vi "Measure JV curve.vi"(4 "Skip pixel?":bool, 6 "Scan settings":T1={"J-V scan"=TRUE, "J-t scan"=FALSE, "Min voltage (V)"=0.0, "Max voltage (V)"=1.4, "Step (V)"=0.01, "Measurement delay (ms)"=10.0, "1st scan FB-SC"=TRUE, "Inverted structure"=FALSE, "Stabilisation time (s)"=0.0, "Stabilisation mode"=0, "Stabilisation value (V or A) "=0.0, "Step time (s)"=1.0, "Integration time"=0, "Repeat light scans"=FALSE, "Stabilisation in the dark?"=FALSE, "J-t Min (V)"=0.0, "J-t Max (V)"=1.4, "J-t Step (V)"=0.01, "Max. power stabilisation"=FALSE, "J-t 1st scan FB-SC"=TRUE, "J-t Inverted structure"=FALSE, "Max power tracking"=FALSE, "Vmp (V)"=0.7, "Total stabilisation time (s)"=100.0, "J-t best pixel only"=0, "Max power best pixel only"=0, "Vmp from J-V scan"=FALSE, "Intensity dependence"=FALSE, "P dep best pixel only"=0, "External quantum efficiency"=FALSE, "EQE best pixel only"=0, "WL min (nm)"=300.0, "WL max (nm)"=900.0, "WL step (nm)"=5.0, "Wait (ms)"=100.0, "No. of repeat scans"=2.0, "Only repeat for best pixel"=0, "Chopper Freq. min (Hz)"=90.0, "Time Constant min (s)"=2.0, "Stabilisation time step (s)"=1.0, "Illumination conditions"=2, "Scan rate min (V/s)"=0.1, "Scan rate max (V/s)"=1.0, "No. of scan rate steps"=1.0, "Scan rate voltage step priority"=FALSE, "Scan rate measurement delay priority"=FALSE, "J-t Illumination conditions"=0, "Chopper Freq. max (Hz)"=200.0, "No. of freq. steps"=1.0, "Time Constant max (s)"=2.0, "No. of t const. steps"=1.0, "White bias min (no. of suns)"=0.1, "White bias max (no. of suns)"=1.0, "No. of white bias steps"=1.0, "Repeat EQE scans"=FALSE, "No. of EQE scans"=2.0, "Max P stab. Specific voltage"=FALSE} {"No. of EQE scans" min=1.0 step=1.0; "No. of white bias steps" min=1.0 step=1.0; "No. of t const. steps" min=1.0 step=1.0; "Time Constant max (s)" items=["0.01s", "0.03s", "0.1s", "0.3s", "1s", "3s"]; "No. of freq. steps" min=1.0 step=1.0; "J-t Illumination conditions" items=["Light only", "Dark only", "Light then dark", "Dark then light"]; "No. of scan rate steps" min=1.0 step=1.0; "Illumination conditions" items=["Light only", "Dark only", "Light then dark", "Dark then light", "Light then dark then light", "Dark then light then dark"]; "Time Constant min (s)" items=["0.01s", "0.03s", "0.1s", "0.3s", "1s", "3s"]; "Only repeat for best pixel" items=["only for best pixel", "for best 2 pixels", "for best 3 pixels", "for best 4 pixels", "for best 5 pixels", "for best 6 pixels", "for best 7 pixels", "for all pixels"]; "No. of repeat scans" min=1.0 step=1.0; "EQE best pixel only" items=["only the best pixel", "the best 2 pixel", "the best 3 pixel", "the best 4 pixel", "the best 5 pixel", "the best 6 pixel", "the best 7 pixel", "all pixels"]; "P dep best pixel only" items=["only the best pixel", "the best 2 pixels", "the best 3 pixels", "the best 4 pixels", "the best 5 pixels", "the best 6 pixels", "the best 7 pixels", "all pixels"]; "Max power best pixel only" items=["only the best pixel", "the best 2 pixels", "the best 3 pixels", "the best 4 pixels", "the best 5 pixels", "the best 6 pixels", "the best 7 pixels", "all pixels"]; "J-t best pixel only" items=["only the best pixel", "the best 2 pixels", "the best 3 pixels", "the best 4 pixels", "the best 5 pixels", "the best 6 pixels", "the best 7 pixels", "all pixels"]; "Integration time" items=["Fast", "Normal", "High Accuracy"]; "Stabilisation mode" items=["V", "I"]; "Measurement delay (ms)" min=10.0}, 7 "Cell details cluster":T3={"Cell Position"=16, "Cell Label"="", "Pixel to measure"=0, "Area (cm^2)"=0.126, "Variable"="", "Variable value"="", "Scan settings in queue"=0, "Light or dark"="", "Measurement type"=""} {"Pixel to measure" items=["All", "1", "2", "3", "4", "5", "6", "7", "8"]}, 8 "Intensity (no. of suns)":string, 9 "Scan rate (V/s)":dbl, 10 "Experiment Title":string, 11 "User Name":string) -> (0 "Log Table":string[][](table), 2 "File path for master log":path, 3 "JV Curve":cluster{"Y":dbl[], "Y":dbl[]}[](graph))   [LabVIEW 2011]
uses:
  TypeDefs/Scan settings.ctl
  TypeDefs/Settings Boolean.ctl
  TypeDefs/NPLC for JV scan.ctl
  <instrlib>/keithley_24xx/Keithley 24XX/Public/Data/Read (Single Point).vi
  <instrlib>/keithley_24xx/Keithley 24XX/Keithley 24XX.lvlib
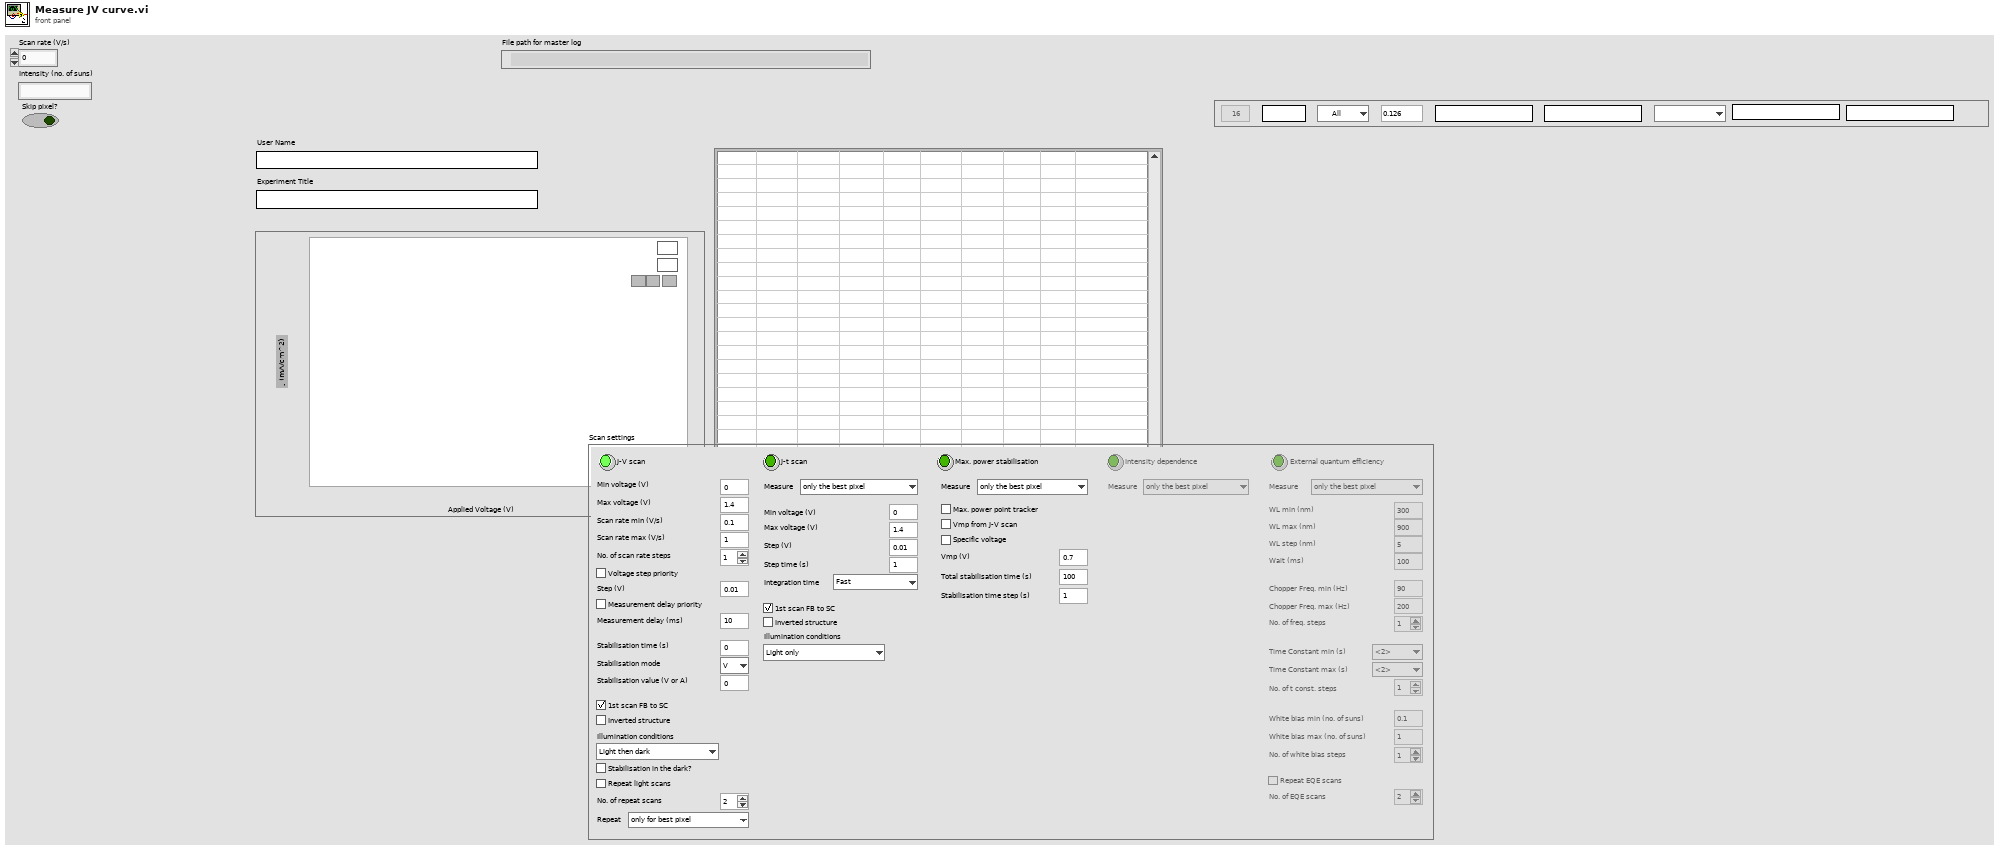
[diagram p1: front panel]
types:
  T1 = typedef "Scan settings.ctl" = cluster{"J-V scan":T2, "J-t scan":bool, "Min voltage (V)":dbl, "Max voltage (V)":dbl, "Step (V)":dbl, "Measurement delay (ms)":dbl, "1st scan FB-SC":bool, "Inverted structure":bool, "Stabilisation time (s)":dbl, "Stabilisation mode":u16, "Stabilisation value (V or A) ":dbl, "Step time (s)":dbl, "Integration time":u16, "Repeat light scans":bool, "Stabilisation in the dark?":bool, "J-t Min (V)":dbl, "J-t Max (V)":dbl, "J-t Step (V)":dbl, "Max. power stabilisation":bool, "J-t 1st scan FB-SC":bool, "J-t Inverted structure":bool, "Max power tracking":bool, "Vmp (V)":dbl, "Total stabilisation time (s)":dbl, "J-t best pixel only":u16, "Max power best pixel only":u16, "Vmp from J-V scan":bool, "Intensity dependence":bool, "P dep best pixel only":u16, "External quantum efficiency":bool, "EQE best pixel only":u16, "WL min (nm)":dbl, "WL max (nm)":dbl, "WL step (nm)":dbl, "Wait (ms)":dbl, "No. of repeat scans":dbl, "Only repeat for best pixel":u16, "Chopper Freq. min (Hz)":dbl, "Time Constant min (s)":dbl, "Stabilisation time step (s)":dbl, "Illumination conditions":u16, "Scan rate min (V/s)":dbl, "Scan rate max (V/s)":dbl, "No. of scan rate steps":dbl, "Scan rate voltage step priority":bool, "Scan rate measurement delay priority":bool, "J-t Illumination conditions":u16, "Chopper Freq. max (Hz)":dbl, "No. of freq. steps":dbl, "Time Constant max (s)":dbl, "No. of t const. steps":dbl, "White bias min (no. of suns)":dbl, "White bias max (no. of suns)":dbl, "No. of white bias steps":dbl, "Repeat EQE scans":bool, "No. of EQE scans":dbl, "Max P stab. Specific voltage":bool}
  T2 = typedef "Settings Boolean.ctl" = bool
  T3 = cluster{"Cell Position":i32, "Cell Label":string, "Pixel to measure":u16, "Area (cm^2)":dbl, "Variable":string, "Variable value":string, "Scan settings in queue":u16, "Light or dark":string, "Measurement type":string}
  T4 = typedef "NPLC for JV scan.ctl" = dbl
  T5 = typedef "imagedata.ctl" = cluster{"image type":i32, "image depth":i32, "image":u8[], "mask":u8[], "colors":u32[], "Rectangle":cluster{"left":i16, "top":i16, "right":i16, "bottom":i16}}
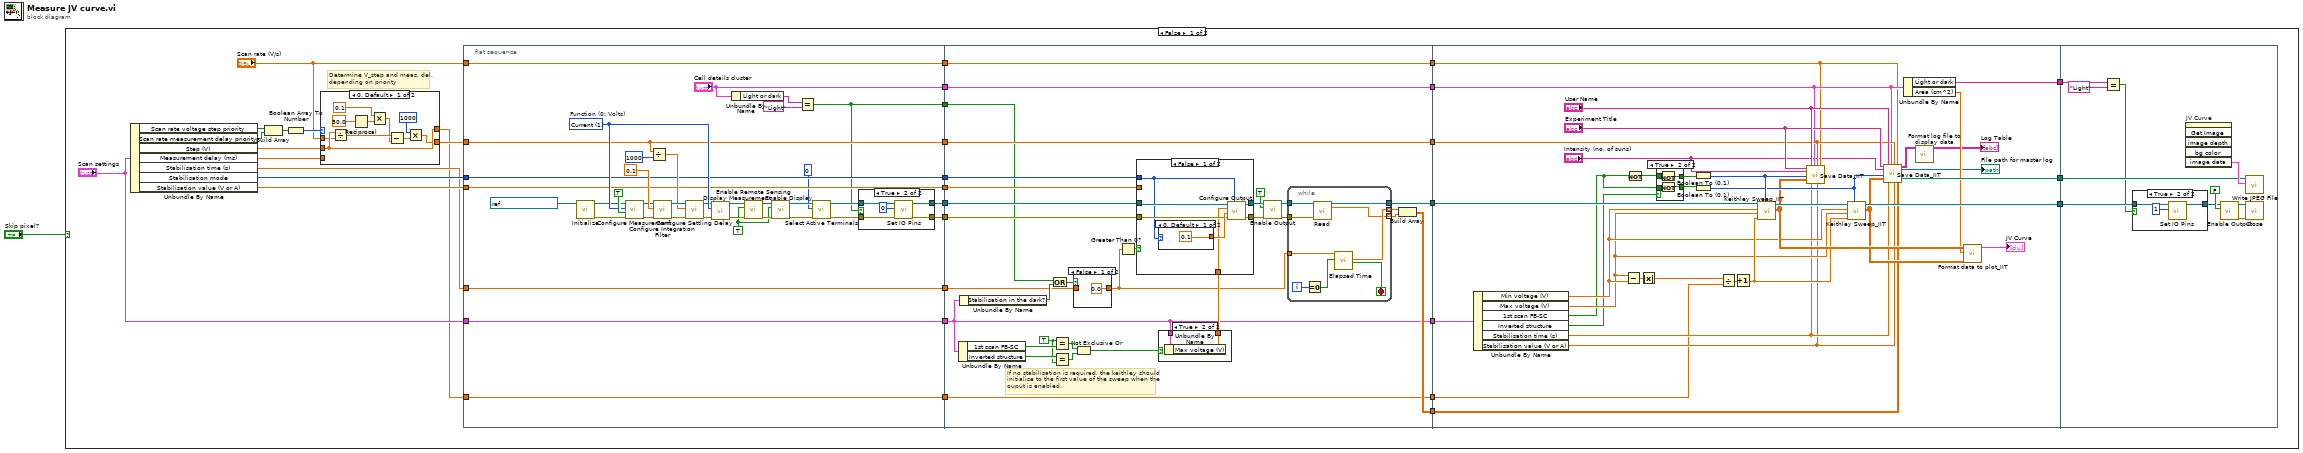
[diagram p0: block diagram]
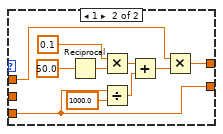
[diagram p2: hidden frame]
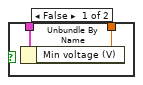
[diagram p5: hidden frame]
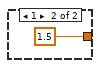
[diagram p6: hidden frame]
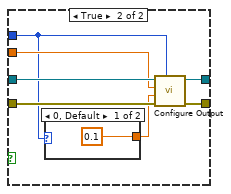
[diagram p7: hidden frame]
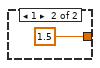
[diagram p8: hidden frame]
diagram:
  n1 = case shown="False" "Skip pixel?" {
    frame False {
      # "Determine V_step and meas. del.\ndepending on priority"
      n2 = Unbundle By Name("Scan settings") -> ("Scan rate voltage step priority"=w9:bool, "Scan rate measurement delay priority"=w8:bool, "Step (V)"=w3:dbl, "Measurement delay (ms)"=w5:dbl, "Stabilisation time (s)"=w11:dbl, "Stabilisation mode"=w13:u16, "Stabilisation value (V or A)"=w14:dbl)
      n3 = Build Array(w9, w8) -> (w10:bool[])
      n4 = Boolean Array To Number(Boolean array=w10) -> (number=w7:u32)
      n5 = case shown="0, Default" w7 {
        tunnel: [w39 w51] -> w6
        tunnel: w5 -> [_ w51]
        tunnel: "Scan rate (V/s)" -> [w36 w47]
        tunnel: [w45 w46] -> w4
        tunnel: w3 -> [w45 _]
        frame 0, Default {
          n6 = Divide(x=w45, y=w36) -> (x/y=w41:dbl)
          n7 = Reciprocal(x=50.0) -> (1/x=w43:dbl)
          n8 = Multiply(x=T4 0.1, y=w43) -> (x*y=w40:T4)
          n9 = Subtract(x=w41, y=w40) -> (x-y=w38:T4)
          n10 = Multiply(x=1000, y=w38) -> (x*y=w39:T4)
        }
        frame 1 {
          n11 = Reciprocal(x=50.0) -> (1/x=w54:dbl)
          n12 = Multiply(x=T4 0.1, y=w54) -> (x*y=w52:T4)
          n13 = Divide(x=w51, y=1000.0) -> (x/y=w49:dbl)
          n14 = Add(x=w52, y=w49) -> (x+y=w48:T4)
          n15 = Multiply(x=w47, y=w48) -> (x*y=w46:T4)
        }
      }
      n16 = flat-sequence {
        tunnel: [w73] -> w35
        tunnel: [w66] -> w34
        tunnel: [w67] -> w33
        tunnel: w14 -> [w73]
        tunnel: [w72] -> w32
        tunnel: w13 -> [w72]
        tunnel: [w71] -> w31
        tunnel: w11 -> [w71]
        tunnel: w6 -> [w70]
        tunnel: [w70] -> w30
        tunnel: [w69] -> w29
        tunnel: "Scan settings" -> [w69]
        tunnel: ["Cell details cluster"] -> w28
        tunnel: [w58] -> w27
        tunnel: [w57] -> w26
        tunnel: w4 -> [w57]
        tunnel: [w56] -> w25
        tunnel: "Scan rate (V/s)" -> [w56]
        tunnel: w35 -> [w119]
        tunnel: w34 -> [w127]
        tunnel: w33 -> [w128]
        tunnel: [w123] -> w24
        tunnel: [w120] -> w23
        tunnel: w32 -> [w116]
        tunnel: w31 -> [w102]
        tunnel: [w118] -> w22
        tunnel: w30 -> [w118]
        tunnel: [w107] -> w21
        tunnel: w29 -> [w107]
        tunnel: [w117] -> w20
        tunnel: w28 -> [w117]
        tunnel: w27 -> [w105]
        tunnel: [w101] -> w19
        tunnel: w26 -> [w101]
        tunnel: [w100] -> w18
        tunnel: w25 -> [w100]
        tunnel: [w192] -> w17
        tunnel: [w185] -> w16
        tunnel: w24 -> [w199]
        tunnel: w23 -> [w184]
        tunnel: w22 -> [w181]
        tunnel: w21 -> [w180]
        tunnel: w20 -> [w174]
        tunnel: [w173] -> w15
        tunnel: w19 -> [w166]
        tunnel: w18 -> [w165]
        tunnel: w17 -> [w210]
        tunnel: w16 -> [w211]
        tunnel: w15 -> [w206]
        frame #0 {
          w74 = TRUE ("Enable Output (T: Enable)")
          w87 = u16 1 items=["Volts", "Current", "Resistance"]  # Function (0: Volts)
          n17 = call <instrlib>:"Initialize.vi"("VISA resource name"=refnum<visa-resource-name> "GPIB0::24::INSTR") -> ("error out"=w77:errorcluster, "VISA resource name out"=w78:refnum<visa-resource-name>)  [unwired: 4 in, 5 out]
          n18 = call <instrlib>:"Configure Measurement.vi"("error in (no error)"=w77, "Enable Auto Range (T:Enable)"=TRUE, "Function (0: Volts)"=w87, "VISA resource name"=w78) -> ("error out"=w80:errorcluster, "VISA resource name out"=w79:refnum<visa-resource-name>)  [unwired: 6 in]
          n19 = Divide(x=w70, y=1000) -> (x/y=w86:T4)
          n20 = call <instrlib>:"Configure Integration Filter.vi"("error in (no error)"=w80, "Measurement Speed (1 PLC)"=T4 0.1, "VISA resource name"=w79) -> ("error out"=w89:errorcluster, "VISA resource name out"=w88:refnum<visa-resource-name>)  [unwired: 7 in]
          n21 = call <instrlib>:"Configure Settling Delay.vi"("error in (no error)"=w89, "Manual Settling Delay (0 sec)"=w86, "VISA resource name"=w88) -> ("error out"=w84:errorcluster, "VISA resource name out"=w83:refnum<visa-resource-name>)  [unwired: 7 in]
          n22 = call <instrlib>:"Display Measurement.vi"("error in (no error)"=w84, "Displayed Measurement (0: Voltage)"=w87, "VISA resource name"=w83) -> ("error out"=w82:errorcluster, "VISA resource name out"=w81:refnum<visa-resource-name>)  [unwired: 7 in]
          n23 = Unbundle By Name("Cell details cluster") -> ("Light or dark"=w65:string)
          n24 = call <instrlib>:"Enable Remote Sensing.vi"("error in (no error)"=w82, "Enable Remote Sensing (T: Enable)"=w74, "VISA resource name"=w81) -> ("error out"=w75:errorcluster, "VISA resource name out"=w76:refnum<visa-resource-name>)  [unwired: 7 in]
          n25 = call <instrlib>:"Enable Display.vi"("error in (no error)"=w75, "Enable Display (T: Enable)"=w74, "VISA resource name"=w76) -> ("error out"=w62:errorcluster, "VISA resource name out"=w63:refnum<visa-resource-name>)  [unwired: 7 in]
          n26 = Equal?(x=w65, y="Light") -> (x = y?=w58:bool)
          n27 = call <instrlib>:"Select Active Terminals.vi"("error in (no error)"=w62, "Active Terminals (0: Front)"=0, "VISA resource name"=w63) -> ("error out"=w60:errorcluster, "VISA resource name out"=w61:refnum<visa-resource-name>)  [unwired: 7 in]
          n28 = case shown="True" w58 {
            tunnel: w61 -> [w94 w98]
            tunnel: w60 -> [w93 w97]
            tunnel: [w94 w96] -> w67
            tunnel: [w93 w95] -> w66
            frame False {
            }
            frame True {
              n29 = call <instrlib>:"Set IO Pins.vi"("error in (no error)"=w97, "Output Pattern (0)"=0, "VISA resource name"=w98) -> ("error out"=w95:errorcluster, "VISA resource name out"=w96:refnum<visa-resource-name>)  [unwired: 7 in]
            }
          }
        }
        frame #1 {
          w112 = TRUE
          # "If no stabilisation is required, the keithley should\ninitialise to the first value of the sweep when the\nouput is enabled."
          n30 = Unbundle By Name(w107) -> ("1st scan FB-SC"=w114:bool, "Inverted structure"=w113:bool)
          n31 = Unbundle By Name(w107) -> ("Stabilisation in the dark?"=w106:bool)
          n32 = Or(x=w105, y=w106) -> (x .or. y?=w104:bool)
          n33 = Equal?(x=w112, y=w114) -> (x = y?=w110:bool)
          n34 = Equal?(x=w113, y=w112) -> (x = y?=w109:bool)
          n35 = case shown="False" w104 {
            tunnel: [0.0 ("Stabilisation time (s)") w132] -> w103
            tunnel: w102 -> [_ w132]
            frame False {
            }
            frame True {
            }
          }
          n36 = Not Exclusive Or(1:w109, 2:w110) -> (0:w108:bool)
          n37 = Greater Than 0?(x=w103) -> (x > 0?=w115:bool)
          n38 = case shown="True" w108 {
            tunnel: w107 -> [w133 w136]
            tunnel: [w134 w135] -> w111
            frame False {
              n39 = Unbundle By Name(w133) -> ("Min voltage (V)"=w134:dbl)
            }
            frame True {
              n40 = Unbundle By Name(w136) -> ("Max voltage (V)"=w135:dbl)
            }
          }
          n41 = case shown="False" w115 {
            tunnel: [w141 w152] -> w130
            tunnel: [w142 w151] -> w129
            tunnel: w128 -> [w139 w150]
            tunnel: w127 -> [w140 w149]
            tunnel: w119 -> [_ w148]
            tunnel: w116 -> [w138 w147]
            tunnel: w111 -> [w137 _]
            frame False {
              n42 = case shown="0, Default" w138 {
                tunnel: [0.1 1.5] -> w143
                frame 0, Default {
                }
                frame 1 {
                }
              }
              n43 = call <instrlib>:"Configure Output.vi"("Source Mode  (0: Voltage)"=w138, "error in (no error)"=w140, "Compliance  Level (0.1)"=w143, "Output Level (0)"=w137, "VISA resource name"=w139) -> ("error out"=w141:errorcluster, "VISA resource name out"=w142:refnum<visa-resource-name>)  [unwired: 5 in]
            }
            frame True {
              n44 = case shown="0, Default" w147 {
                tunnel: [0.1 1.5] -> w146
                frame 0, Default {
                }
                frame 1 {
                }
              }
              n45 = call <instrlib>:"Configure Output.vi"("Source Mode  (0: Voltage)"=w147, "error in (no error)"=w149, "Compliance  Level (0.1)"=w146, "Output Level (0)"=w148, "VISA resource name"=w150) -> ("error out"=w152:errorcluster, "VISA resource name out"=w151:refnum<visa-resource-name>)  [unwired: 5 in]
            }
          }
          n46 = call <instrlib>:"Enable Output.vi"("error in (no error)"=w130, "Enable Output (T: Enable)"=TRUE ("Output (Off)"), "VISA resource name"=w129) -> ("error out"=w124:errorcluster, "VISA resource name out"=w125:refnum<visa-resource-name>)  [unwired: 7 in]
          n47 = while {
            tunnel: w125 -> [w163]
            tunnel: w124 -> [w162]
            tunnel: [w161] -> w123
            tunnel: [w159] -> w122 mode=indexing
            tunnel: [w158] -> w121 mode=indexing
            tunnel: w103 -> [w155]
            i -> [w157]
            stop <- w160 stop-if-true
            n48 = Equal To 0?(x=w157) -> (x = 0?=w156:bool)
            n49 = call-poly <instrlib>:"Read.vi"("VISA resource name"=w163, "error in (no error)"=w162) -> ("VISA resource name out"=w161:refnum<visa-resource-name>, "Current"=w158:sgl)  [unwired: 7 in, 5 out]
            n50 = call "Elapsed Time"("Time Target (s)"=w155, "Reset"=w156) -> ("Elapsed Time (s)"=w159:dbl, "Time has Elapsed"=w160:bool)  [unwired: 10 in, 6 out]
          }
          n51 = Build Array(w122, w121) -> (w120:dbl[][])
        }
        frame #2 {
          n52 = Unbundle By Name(w180) -> ("Min voltage (V)"=w179:dbl, "Max voltage (V)"=w178:dbl, "1st scan FB-SC"=w168:bool, "Inverted structure"=w177:bool, "Stabilisation time (s)"=w176:dbl, "Stabilisation value (V or A)"=w175:dbl)
          n53 = Subtract(x=w178, y=w179) -> (x-y=w197:dbl)
          n54 = Not(x=w168) -> (.not. x?=w169:bool)
          n55 = Absolute Value(x=w197) -> (abs(x)=w198:dbl)
          n56 = case shown="True" w177 {
            tunnel: [w201 w205] -> w187
            tunnel: [w200 w204] -> w186
            tunnel: w168 -> [w200 w203]
            tunnel: w169 -> [w201 w202]
            frame False {
            }
            frame True {
              n57 = Not(x=w202) -> (.not. x?=w205:bool)
              n58 = Not(x=w203) -> (.not. x?=w204:bool)
            }
          }
          n59 = Boolean To (0,1)(Boolean=w187) -> (0, 1=w195:i16)
          n60 = Boolean To (0,1)(Boolean=w186) -> (0, 1=w193:i16)
          n61 = Divide(x=w198, y=w166) -> (x/y=w189:T4)
          n62 = Increment(x=w189) -> (x+1=w188:T4)
          n63 = call "Keithley Sweep_IIT.vi"("Sweep Direction"=w195, "Number of Points"=w188, "Maximum Amplitude"=w178, "Minimum Amplitude"=w179, "VISA resource name out 2"=w199) -> ("Data Array"=w191:dbl[][], "VISA resource name out"=w194:refnum<visa-resource-name>)  [unwired: 2 in, 1 out]
          n64 = call "Save Data_IIT.vi"("Experiment Indicator"="Experiment Title", "Intensity (no. of suns)"="Intensity (no. of suns)", "Scan direction"=w195, "Data Array"=w191, "Username"="User Name", "Stabilisation time (ms)"=w176, "Cell details cluster"=w174, "Measurement Delay (ms)"=w181, "Stabilisation level \n(A or V depending on mode)"=w175, "Scan rate (V/s)"=w165) -> ()  [unwired: 6 in, 4 out]
          n65 = call "Keithley Sweep_IIT.vi"("Sweep Direction"=w193, "Number of Points"=w188, "Maximum Amplitude"=w178, "Minimum Amplitude"=w179, "VISA resource name out 2"=w194) -> ("Data Array"=w190:dbl[][], "VISA resource name out"=w192:refnum<visa-resource-name>)  [unwired: 2 in, 1 out]
          n66 = call "Save Data_IIT.vi"("Experiment Indicator"="Experiment Title", "Intensity (no. of suns)"="Intensity (no. of suns)", "Scan direction"=w193, "Data Array"=w190, "Username"="User Name", "Stabilisation time (ms)"=w176, "Cell details cluster"=w174, "Measurement Delay (ms)"=w181, "Stabilisation level \n(A or V depending on mode)"=w175, "Scan rate (V/s)"=w165, "Stabilisation Data"=w184) -> ("Master Log"=w171:string[][], "File path for master log"=→"File path for master log":path, "File path for JV image"=w185:path)  [unwired: 5 in, 1 out]
          n67 = Unbundle By Name(w174) -> ("Light or dark"=w173:string, "Area (cm^2)"=w172:dbl)
          n68 = call "Format log file to display data.vi"("Master Log"=w171) -> ("Formatted table"=→"Log Table":string[][])  [unwired: 10 in]
          n69 = call "Format data to plot_IIT.vi"("Data Array 2"=w190, "Device Area (cm^2)"=w172, "Data Array"=w191) -> ("JV Curve"=→"JV Curve":cluster{"Y":dbl[], "Y":dbl[]}[])  [unwired: 8 in]
        }
        frame #3 {
          n70 = Equal?(x=w206, y="Light") -> (x = y?=w207:bool)
          n71 = case shown="True" w207 {
            tunnel: w210 -> [w216 w218]
            tunnel: [w216 w217] -> w209
            frame False {
            }
            frame True {
              n72 = call <instrlib>:"Set IO Pins.vi"("Output Pattern (0)"=1, "VISA resource name"=w218) -> ("VISA resource name out"=w217:refnum<visa-resource-name>)  [unwired: 8 in, 1 out]
            }
          }
          n73 = invoke on="JV Curve" class="XYGraph (strict)" method="Get Image"() -> ("image data"=w212:T5)  [unwired: 6 in, 5 out]
          n74 = call <instrlib>:"Enable Output.vi"("Enable Output (T: Enable)"=FALSE ("Output (Off)"), "VISA resource name"=w209) -> ("error out"=w214:errorcluster, "VISA resource name out"=w215:refnum<visa-resource-name>)  [unwired: 8 in]
          n75 = call <vilib>:"Write JPEG File.vi"("image data"=w212, "path to JPEG file"=w211) -> ()  [unwired: 8 in, 2 out]
          n76 = call <instrlib>:"Close.vi"("error in (no error)"=w214, "VISA resource name"=w215) -> ()  [unwired: 9 in, 1 out]
        }
      }
    }
    frame True {
    }
  }
